vi "GPIB Command Line.vi"() -> ()   [LabVIEW 2023]
doc: "A command-line interface that allows you to send commands and read responses from any GPIB instrument attached to the system."
uses:
  instrument list.ctl
panel:
  out "timeout":bool
  in  "instrument":T1=11 items=["photon counter"=23, "pulse generator"=10, "lock-in"=9, "spectrometer"=1, "microwave generator"=19, "function generator"=11, "laser power controller"=8, "other"=0]
  in  "GPIB address":u16=11
  in  "send":bool
  in  "exit":bool
  out "received data":string
  in  "write string":string="*IDN?"
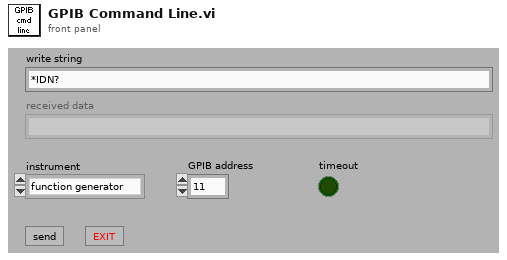
[diagram p1: front panel]
types:
  T1 = typedef "instrument list.ctl" = u16
  T2 = typedef "LVStringsAndValuesArrayTypeDef_U16.ctl" = cluster{"String":string, "Value":u16}[]
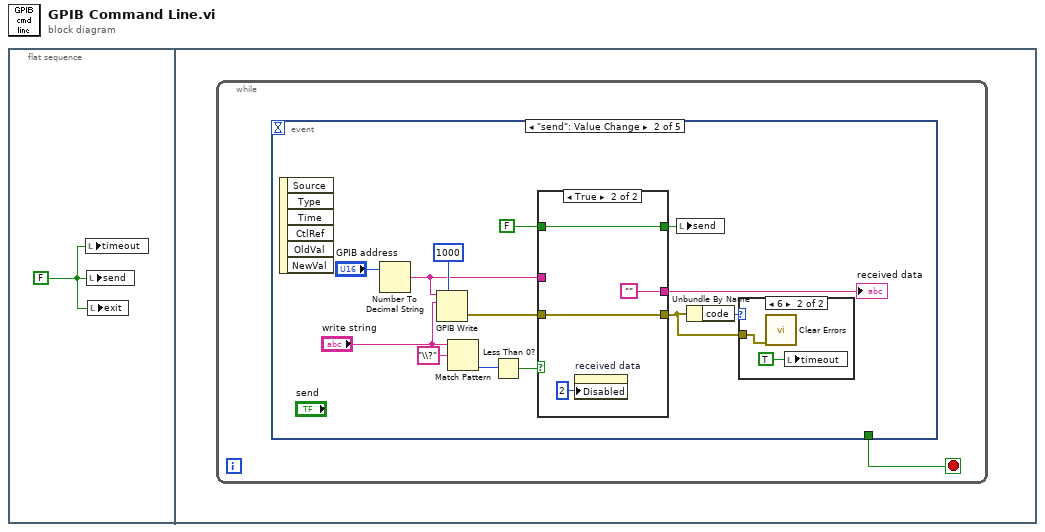
[diagram p0: block diagram]
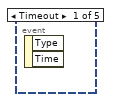
[diagram p2: hidden frame]
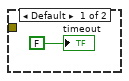
[diagram p3: hidden frame]
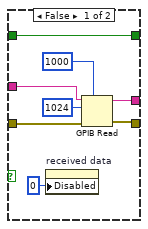
[diagram p4: hidden frame]
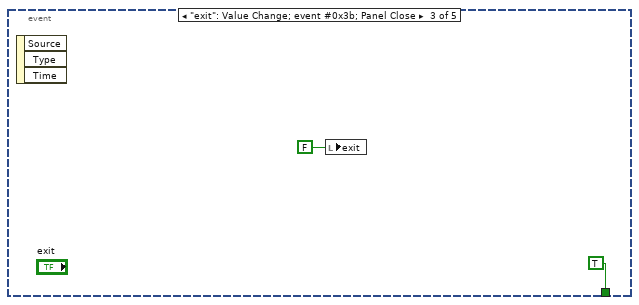
[diagram p5: hidden frame]
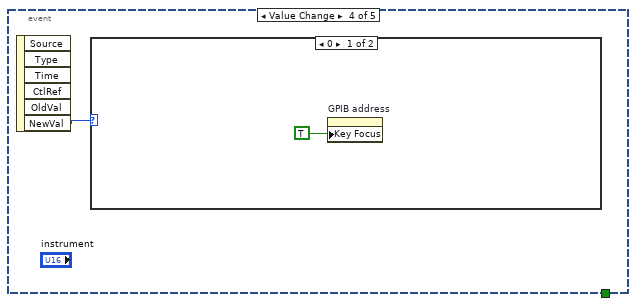
[diagram p6: hidden frame]
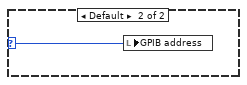
[diagram p7: hidden frame]
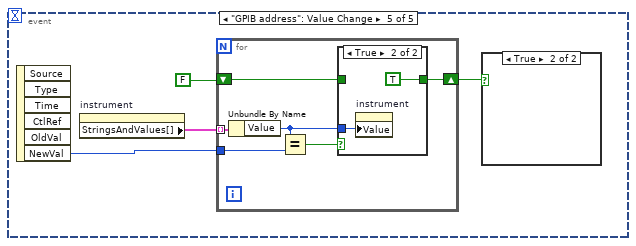
[diagram p8: hidden frame]
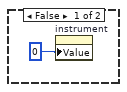
[diagram p9: hidden frame]
diagram:
  n1 = flat-sequence {
    frame #0 {
      w1 = FALSE ("exit")
      n2 = local write "timeout"(w1) -> ()
      n3 = local write "send"(w1) -> ()
      n4 = local write "exit"(w1) -> ()
    }
    frame #1 {
      n5 = while {
        stop <- w2 stop-if-true
        n6 = event shown="[1] \"send\": Value Change" {
          selector: _ -> [_ _ _ _ _]
          dyn-events: _ -> [_ _ _ _ _]
          timeout: _ -> [_ _ _ _ _]
          tunnel: [_ _ TRUE _ _] -> w2
          event Timeout {
            n7 = event-data() -> ()  [unwired: 3 out]
          }
          event "send": Value Change {
            n8 = event-data() -> ()  [unwired: 7 out]
            n9 = Number To Decimal String(number="GPIB address") -> (decimal integer string=w7:string)  [unwired: 1 out]
            n10 = GPIB Write(0:w7, 1:"write string", 4:1000 ("timeout ms (488.2 global)")) -> (6:w15:errorcluster)  [unwired: 1 in, 2 out]
            n11 = Match Pattern(string="write string", regular expression="\\?") -> (offset past match=w11:i32)  [unwired: 4 out]
            n12 = Less Than 0?(x=w11) -> (x < 0?=w10:bool)
            n13 = case shown="True" w10 {
              tunnel: w15 -> [w26 w28]
              tunnel: w7 -> [w25 _]
              tunnel: [w22 ""] -> w9
              tunnel: [w20 w28] -> w6
              tunnel: FALSE ("send") -> [w19 w27]
              tunnel: [w19 w27] -> w3
              frame False {
                n14 = property on="received data" class="Str"("Disabled"=u8 0) -> ()  [unwired: 2 in, 2 out]
                n15 = GPIB Read(0:w25, 1:1024 ("byte count"), 3:w26, 4:1000 ("timeout ms (488.2 global)")) -> (5:w22:string, 7:w20:errorcluster)  [unwired: 2 out]
              }
              frame True {
                n16 = property on="received data" class="Str"("Disabled"=u8 2) -> ()  [unwired: 2 in, 2 out]
              }
            }
            "received data" <- w9
            n17 = local write "send"(w3) -> ()
            n18 = Unbundle By Name(w6) -> ("code"=w5:i32)
            n19 = case shown="6" w5 {
              tunnel: w6 -> [_ w18]
              frame Default {
                "timeout" <- FALSE ("timeout")
              }
              frame 6 {
                n20 = call <vilib>:"Clear Errors.vi"("error in (no error)"=w18) -> ()  [unwired: 1 in, 6 out]
                n21 = local write "timeout"(TRUE ("timeout")) -> ()
              }
            }
          }
          event "exit": Value Change; event #0x3b; Panel Close {
            n22 = event-data() -> ()  [unwired: 4 out]
            n23 = local write "exit"(FALSE ("exit")) -> ()
          }
          event Value Change {
            n24 = event-data() -> ("NewVal"=w33:T1)  [unwired: 6 out]
            n25 = case shown="0" w33 {
              selector: w33 -> [_ w35]
              frame 0 {
                n26 = property on="GPIB address" class="DigNum (strict)"("Key Focus"=TRUE) -> ()  [unwired: 2 in, 2 out]
              }
              frame Default {
                n27 = local write "GPIB address"(w35) -> ()
              }
            }
          }
          event "GPIB address": Value Change {
            n28 = event-data() -> ("NewVal"=w38:u16)  [unwired: 6 out]
            n29 = property on="instrument" class="Ring (strict)"() -> ("StringsAndValues[]"=w39:T2)  [unwired: 2 in, 2 out]
            n30 = for {
              tunnel: w39 -> [w44] mode=indexing
              tunnel: w38 -> [w46]
              shift-right: [w41] -> w36
              shift-left: FALSE -> [w42]
              n31 = Unbundle By Name(w44) -> ("Value"=w43:u16)
              n32 = Equal?(x=w43, y=w46) -> (x = y?=w45:bool)
              n33 = case shown="True" w45 {
                tunnel: w43 -> [_ w49]
                tunnel: w42 -> [w47 _]
                tunnel: [w47 TRUE] -> w41
                frame False {
                }
                frame True {
                  n34 = property on="instrument" class="Ring (strict)"("Value"=w49) -> ()  [unwired: 2 in, 2 out]
                }
              }
            }
            n35 = case shown="True" w36 {
              frame False {
                n36 = property on="instrument" class="Ring (strict)"("Value"=0) -> ()  [unwired: 2 in, 2 out]
              }
              frame True {
              }
            }
          }
        }
      }
    }
  }
